vi "FPGAvi.vi"() -> ()   [LabVIEW 2017]
uses:
  <vilib>/Platform/TimedLoop/XDataNode/wakeup.ctl
  <vilib>/Platform/TimedLoop/XDataNode/XDNodeRunTimeDep.lvlib
  <vilib>/Platform/TimedLoop/XDataNode/nitl_modes.ctl
  <vilib>/Platform/TimedLoop/XDataNode/timing_clust.ctl
  <vilib>/Platform/TimedLoop/XDataNode/XDataNode.xnode
  <vilib>/eio/EIONode/EIONode.xnode
  <vilib>/rvi/eio/common/nirviEmuTemplateMethod_errors.vi
  <vilib>/rvi/occurrence/nirviOccurrence.lvlib
  Control/GV DO delay.vi
  Control/GV FIFO timeout.vi
  Control/GV trigger delay.vi
  Detector/GV gated pixelclock change.vi
  Detector/GV frameclock.vi
  Detector/GV framegate.vi
  Detector/GV PMT sim.vi
  Detector/GV frame counter.vi
panel:
  in  "Pockels1_EnableManualControl":bool
  in  "FlushTrigger":bool
  in  "NlinesPerFramePlusSkips":u16
  in  "LineclockInputSelector":u8
  in  "PhotoncounterInputSelector":u8
  in  "NlinesPerFrame":u16
  in  "LinegateTrigger":bool
  in  "Shutter 2":bool
  in  "Shutter 1":bool
  in  "EnableFIFO":bool
  in  "RS_voltage":i16
  in  "RS_ON_OFF":bool
  in  "VT_NC":bool
  in  "VT_forward":bool
  in  "VT_back":bool
  in  "VT_start":bool
  in  "SyncAODOtoLinegate_tick":u16
  in  "NlinesAll":u16=1
  in  "Pulse sequence":bool[](array[boolean])=[TRUE, FALSE, FALSE, FALSE, FALSE, FALSE, FALSE, FALSE, FALSE, FALSE, FALSE, FALSE, FALSE, FALSE, FALSE, FALSE, FALSE, FALSE, FALSE, FALSE]
  in  "Nchannels":u16=4
  in  "FIFOtimeout_tick":u16=100
  in  "FIFOINtrigger":bool
  in  "SyncDOtoAOtick":u16=296
  # "RESONANT\nSCANNER"
  # "POCKELS #1"
  # "VIBRATOME"
  # "SHUTTERS"
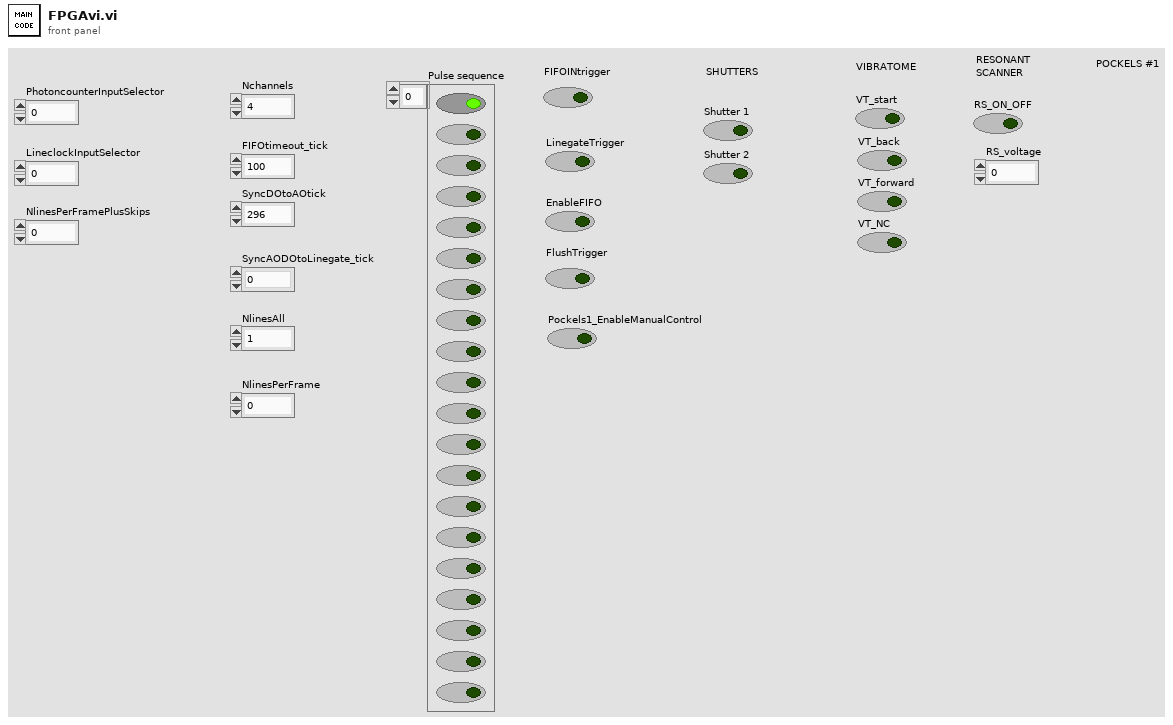
[diagram p1: front panel]
types:
  T1 = typedef "XDNodeRunTimeDep.lvlib/timing_clust.ctl" = cluster{"Expected End [f-1]":u64, "Actual End [f-1]":u64, "Finished Late? [f-1]":bool, "Expected End [i-1]":u64, "Actual End [i-1]":u64, "Finished Late? [i-1]":bool, "Expected Start [i]":u64, "Actual Start [i]":u64, "Expected Start [f]":u64, "Actual Start [f]":u64, "Source Name":string, "Structure Name":string, "Period":i64, "Deadline":i64, "Offset":i64, "Start":i64, "Priority":i32, "Timeout":i32, "Mode":T2, "Wakeup Reason":T3, "Error":errorcluster, "Source Type":string, "Secondary Source Type":string, "Global End Time":u64, "Global Start Time":u64, "Frame Duration":u64, "Iteration Duration":u64, "Assigned CPU":i32, "I/O Scan Engine Mode":u32}
  T2 = typedef "XDNodeRunTimeDep.lvlib/nitl_modes.ctl" = enum32{"No Change", "Process missed periods, maintain original phase", "Discard missed periods, maintain original phase", "Process missed periods, ignore original phase", "Discard missed periods, ignore original phase"}
  T3 = typedef "XDNodeRunTimeDep.lvlib/wakeup.ctl" = enum32{"Normal", "Aborted", "Asynchronous wakeup", "Timing source error", "Timed loop error", "Timeout"}
  T4 = cluster{"Pixelclock change":bool, "Lineclock":bool}
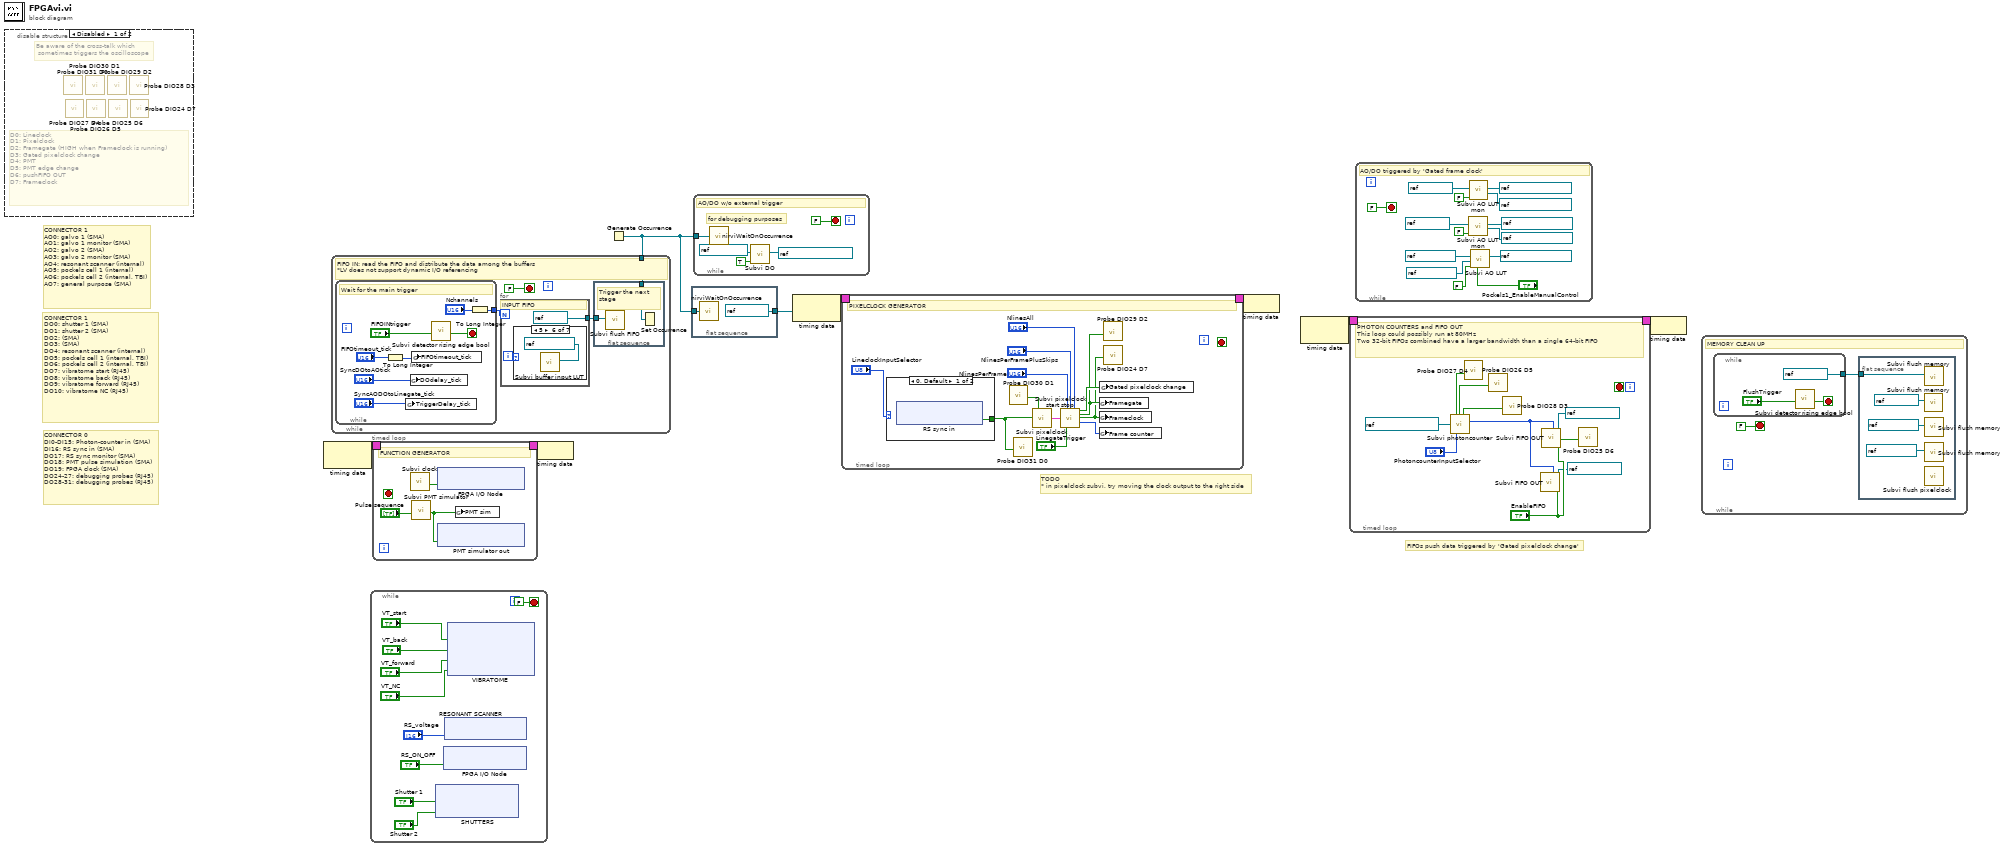
[diagram p0: block diagram]
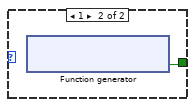
[diagram p2: hidden frame]
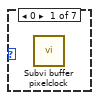
[diagram p4: hidden frame]
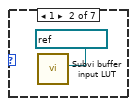
[diagram p5: hidden frame]
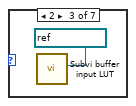
[diagram p6: hidden frame]
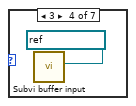
[diagram p7: hidden frame]
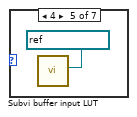
[diagram p8: hidden frame]
diagram:
  # "TODO\n* in pixelclock subvi, try moving the clock output to the right side"
  # "FIFOs push data triggered by 'Gated pixelclock change'"
  # "CONNECTOR 0\nDI0-DI15: Photon-counter in (SMA)\nDI16: RS sync in (SMA)\nDO17: RS sync monitor (SMA)\nDO18: PMT pulse simulation (SMA)\nDO19: FPGA clock (SMA)\nDO24-27: debugging probes (RJ45)\nDO28-31: debugging probes (RJ45)"
  # "CONNECTOR 1\nDO0: shutter 1 (SMA)\nDO1: shutter 2 (SMA)\nDO2: (SMA)\nDO3: (SMA)\nDO4: resonant scanner (internal)\nDO5: pockels cell 1 (internal, TBI)\nDO6: pockels cell 2 (internal, TBI)\nDO7: vibratome start (RJ45)\nDO8: vibratome back (RJ45)\nDO9: vibratome forward (RJ45)\nDO10: vibratome NC (RJ45)"
  # "CONNECTOR 1\nAO0: galvo 1 (SMA)\nAO1: galvo 1 monitor (SMA)\nAO2: galvo 2 (SMA)\nAO3: galvo 2 monitor (SMA)\nAO4: resonant scanner (internal)\nAO5: pockels cell 1 (internal)\nAO6: pockels cell 2 (internal, TBI)\nAO7: general purpose (SMA)"
  n1 = disable-structure shown="Disabled" {
    frame Disabled {
      # "D0: Lineclock\nD1: Pixelclock\nD2: Framegate (HIGH when Frameclock is running)\nD3: Gated pixelclock change\nD4: PMT\nD5: PMT edge change\nD6: pushFIFO OUT\nD7: Frameclock"
      # "Be aware of the cross-talk which\n sometimes triggers the oscilloscope"
      n2 = call "Probe DIO31 D0.vi"() -> ()  [unwired: 12 in]
      n3 = call "Probe DIO27 D4.vi"() -> ()  [unwired: 12 in]
      n4 = call "Probe DIO30 D1.vi"() -> ()  [unwired: 12 in]
      n5 = call "Probe DIO26 D5.vi"() -> ()  [unwired: 12 in]
      n6 = call "Probe DIO29 D2.vi"() -> ()  [unwired: 12 in]
      n7 = call "Probe DIO25 D6.vi"() -> ()  [unwired: 12 in]
      n8 = call "Probe DIO28 D3.vi"() -> ()  [unwired: 12 in]
      n9 = call "Probe DIO24 D7.vi"() -> ()  [unwired: 12 in]
    }
    frame Enabled {
    }
  }
  n10 = node-c288() -> (w8:T1)  [unwired: 1 in]
  n11 = while {
    stop <- FALSE stop-if-true
    n12 = xnode "SHUTTERS"("Connector1/DIO0"="Shutter 1", "Connector1/DIO1"="Shutter 2") -> ()  [unwired: 2 in, 2 out]
    n13 = xnode "FPGA I/O Node"("Connector1/DIO4"="RS_ON_OFF") -> ()  [unwired: 1 in, 1 out]
    n14 = xnode "RESONANT SCANNER"("Connector1/AO4"="RS_voltage") -> ()  [unwired: 1 in, 1 out]
    n15 = xnode "VIBRATOME"("Connector1/DIO7"="VT_start", "Connector1/DIO8"="VT_back", "Connector1/DIO9"="VT_forward", "Connector1/DIO10"="VT_NC") -> ()  [unwired: 4 in, 4 out]
  }
  n16 = timed-loop {
    timing: w8 -> [_]
    timing-out: [_] -> w7
    stop <- _ stop-if-true
    # "FUNCTION GENERATOR"
    n17 = call "Subvi clock.vi"() -> ("Output"=w20:bool)  [unwired: 11 in]
    n18 = call "Subvi PMT simulator.vi"("Pulse sequence"="Pulse sequence") -> ("output"=w18:bool)  [unwired: 10 in]
    n19 = xnode "FPGA I/O Node"("Connector0/DIO19"=w20) -> ()  [unwired: 1 in, 1 out]
    n20 = xnode ("PMT simulator out")("Connector0/DIO18"=w18) -> ()  [unwired: 1 in, 1 out]
    n21 = global write "GV PMT sim.vi" "PMT sim"(w18) -> ()
  }
  n22 = node-c288(w7) -> ()
  n23 = Generate Occurrence() -> (w1:refnum<k4>)
  n24 = while {
    tunnel: w1 -> [w23]
    stop <- FALSE stop-if-true
    # "FIFO IN: read the FIFO and distribute the data among the buffers\n*LV does not support dynamic I/O referencing"
    n25 = while {
      tunnel: [w36] -> w25
      stop <- w43 stop-if-true
      # "Wait for the main trigger"
      n26 = To Long Integer(number="FIFOtimeout_tick") -> (32bit integer=w37:i32)
      n27 = global write "GV trigger delay.vi" "TriggerDelay_tick"("SyncAODOtoLinegate_tick") -> ()
      n28 = global write "GV DO delay.vi" "DOdelay_tick"("SyncDOtoAOtick") -> ()
      n29 = global write "GV FIFO timeout.vi" "FIFOtimeout_tick"(w37) -> ()
      n30 = call "Subvi detector rising edge bool.vi"("Input"="FIFOINtrigger") -> ("Output"=w43:bool)  [unwired: 10 in]
      n31 = To Long Integer(number="Nchannels") -> (32bit integer=w36:i32)
    }
    n32 = for {
      N: w25 -> [_]
      tunnel: [refnum<k21> "FIFO IN" ("FIFO In")] -> w24
      i -> [w30]
      # "INPUT FIFO"
      n33 = case shown="5" w30 {
        frame 0 {
          n34 = call "Subvi buffer pixelclock.vi"() -> ()  [unwired: 12 in]
        }
        frame 1 {
          n35 = call "Subvi buffer input LUT.vi"("Buffer"=refnum<k21> "GALVO1") -> ()  [unwired: 11 in]
        }
        frame 2 {
          n36 = call "Subvi buffer input LUT.vi"("Buffer"=refnum<k21> "GALVO2") -> ()  [unwired: 11 in]
        }
        frame 3 {
          n37 = call "Subvi buffer input.vi"("Buffers"=refnum<k21> "DOdebug" ("FIFO In")) -> ()  [unwired: 11 in]
        }
        frame 4 {
          n38 = call "Subvi buffer input LUT.vi"("Buffer"=refnum<k21> "POCKELS1") -> ()  [unwired: 11 in]
        }
        frame 5 {
          n39 = call "Subvi buffer input LUT.vi"("Buffer"=refnum<k21> "SCALING1") -> ()  [unwired: 11 in]
        }
        frame -1, Default {
        }
      }
    }
    n40 = flat-sequence {
      tunnel: w24 -> [w28]
      tunnel: w23 -> [w27]
      frame #0 {
        # "Trigger the next stage"
        n41 = call "Subvi flush FIFO.vi"("FIFO In"=w28) -> ()  [unwired: 10 in]
        n42 = Set Occurrence(w27) -> ()
      }
    }
  }
  n43 = flat-sequence {
    tunnel: w1 -> [w45]
    tunnel: [refnum<k21> "160MHz" ("Source Name")] -> w2
    frame #0 {
      n44 = call <vilib>:"nirviWaitOnOccurrence.vi"("occurrence"=w45) -> ()  [unwired: 4 in, 1 out]
    }
  }
  n45 = while {
    tunnel: w1 -> [w49]
    stop <- FALSE stop-if-true
    # "for debugging purposes"
    # "AO/DO w/o external trigger"
    n46 = call <vilib>:"nirviWaitOnOccurrence.vi"("occurrence"=w49) -> ()  [unwired: 4 in, 1 out]
    n47 = call "Subvi DO.vi"("DO"=refnum<k21> "Connector1/DIO3", "Ext trigger"=TRUE ("Ext trig enable"), "FIFO In"=refnum<k21> "DOdebug") -> ()  [unwired: 9 in]
  }
  n48 = node-c288(w2) -> (w4:T1)
  n49 = timed-loop {
    timing: w4 -> [_]
    timing-out: [_] -> w3
    stop <- _ stop-if-true
    # "PIXELCLOCK GENERATOR"
    n50 = case shown="0, Default" "LineclockInputSelector" {
      tunnel: [w63 w64] -> w59
      frame 0, Default {
        n51 = xnode "RS sync in"() -> ("Connector0/DIO16"=w63:bool)  [unwired: 1 in, 1 out]
      }
      frame 1 {
        n52 = xnode "Function generator"() -> ("Connector0/DIO17"=w64:bool)  [unwired: 1 in, 1 out]
      }
    }
    n53 = call "Probe DIO31 D0.vi"("D0"=w59) -> ()  [unwired: 11 in]
    n54 = call "Subvi pixelclock.vi"("Lineclock"=w59) -> ("Pixelclock"=w62:bool, "Pixelclock/Lineclock"=w56:T4)  [unwired: 13 in]
    n55 = call "Probe DIO30 D1.vi"("D1"=w62) -> ()  [unwired: 11 in]
    n56 = call "Subvi pixelclock start stop.vi"("Nlines per frame"="NlinesPerFrame", "Nlines per frame plus skips"="NlinesPerFramePlusSkips", "Nlines all"="NlinesAll", "Pixelclock/Lineclock"=w56, "Linegate trigger"="LinegateTrigger") -> ("Gated pixelclock change"=w58:bool, "Framegate"=w57:bool, "Frameclock"=w52:bool, "Frame counter"=w51:u8)  [unwired: 7 in]
    n57 = global write "GV framegate.vi" "Framegate"(w57) -> ()
    n58 = global write "GV frameclock.vi" "Frameclock"(w52) -> ()
    n59 = global write "GV frame counter.vi" "Frame counter"(w51) -> ()
    n60 = global write "GV gated pixelclock change.vi" "Gated pixelclock change"(w58) -> ()
    n61 = call "Probe DIO29 D2.vi"("D2"=w57) -> ()  [unwired: 11 in]
    n62 = call "Probe DIO24 D7.vi"("D7"=w52) -> ()  [unwired: 11 in]
  }
  n63 = node-c288(w3) -> ()
  n64 = node-c288() -> (w6:T1)  [unwired: 1 in]
  n65 = timed-loop {
    timing: w6 -> [_]
    timing-out: [_] -> w5
    stop <- _ stop-if-true
    # "PHOTON COUNTERS and FIFO OUT\nThis loop could possibly run at 80MHz\nTwo 32-bit FIFOs combined have a larger bandwidth than a single 64-bit FIFO"
    n66 = call "Subvi photoncounter.vi"("DI channel"=refnum<k21> "Connector0/DIO0", "Photoncounter input selector"="PhotoncounterInputSelector") -> ("PMT mon"=w68:bool, "PMT edge change mon"=w69:bool, "Gated pixelclock change mon"=w70:bool, "Count"=w75:u8)  [unwired: 10 in]
    n67 = call "Probe DIO27 D4.vi"("D4"=w68) -> ()  [unwired: 11 in]
    n68 = call "Probe DIO26 D5.vi"("D5"=w69) -> ()  [unwired: 11 in]
    n69 = call "Probe DIO28 D3.vi"("D3"=w70) -> ()  [unwired: 11 in]
    n70 = call "Subvi FIFO OUT.vi"("Enable FIFO"="EnableFIFO", "FIFO OUT"=refnum<k21> "FIFO OUT b", "number 1"=w75) -> ()  [unwired: 8 in, 1 out]
    n71 = call "Subvi FIFO OUT.vi"("Enable FIFO"="EnableFIFO", "FIFO OUT"=refnum<k21> "FIFO OUT a", "number 1"=w75) -> ("Push FIFO OUT mon"=w67:bool)  [unwired: 8 in]
    n72 = call "Probe DIO25 D6.vi"("D6"=w67) -> ()  [unwired: 11 in]
  }
  n73 = while {
    stop <- FALSE stop-if-true
    # "AO/DO triggered by 'Gated frame clock'"
    n74 = call "Subvi AO LUT mon.vi"("mon"=refnum<k21> "Connector1/AO3" ("AO mon"), "AO"=refnum<k21> "Connector1/AO2", "Ext trigger"=FALSE ("Ext trig enable"), "FIFO In"=refnum<k21> "GALVO2") -> ()  [unwired: 7 in]
    n75 = call "Subvi AO LUT mon.vi"("mon"=refnum<k21> "Connector1/AO1" ("AO mon"), "AO"=refnum<k21> "Connector1/AO0", "Ext trigger"=FALSE, "FIFO In"=refnum<k21> "GALVO1") -> ()  [unwired: 7 in]
    n76 = call "Subvi AO LUT.vi"("AO"=refnum<k21> "Connector1/AO5", "EnableManualControl"="Pockels1_EnableManualControl", "Ext trigger"=FALSE ("Ext trig enable"), "Scaling Factor"=refnum<k21> "SCALING1", "FIFO In"=refnum<k21> "POCKELS1") -> ()  [unwired: 6 in]
  }
  n77 = node-c288(w5) -> ()
  n78 = while {
    stop <- FALSE stop-if-true
    # "MEMORY CLEAN UP"
    n79 = while {
      tunnel: [refnum<k21> "GALVO1" ("Memory In")] -> w93
      stop <- w97 stop-if-true
      n80 = call "Subvi detector rising edge bool.vi"("Input"="FlushTrigger") -> ("Output"=w97:bool)  [unwired: 10 in]
    }
    n81 = flat-sequence {
      tunnel: w93 -> [w99]
      frame #0 {
        n82 = call "Subvi flush memory.vi"("Memory In"=refnum<k21> "GALVO2") -> ()  [unwired: 10 in]
        n83 = call "Subvi flush memory.vi"("Memory In"=w99) -> ()  [unwired: 10 in]
        n84 = call "Subvi flush memory.vi"("Memory In"=refnum<k21> "POCKELS1") -> ()  [unwired: 10 in]
        n85 = call "Subvi flush memory.vi"("Memory In"=refnum<k21> "SCALING1") -> ()  [unwired: 10 in]
        n86 = call "Subvi flush pixelclock.vi"() -> ()  [unwired: 12 in]
      }
    }
  }
